vi "SetGas.vi"(7 "Timeout (ms)":u32=2000, 8 "Error In":errorcluster, 10 "Gas":T1, 11 "Sierra M100 In":refnum<visa-resource-name>) -> (0 "Error Out":errorcluster, 2 "Set?":bool, 3 "Sierra M100 Out":refnum<visa-resource-name>)   [LabVIEW 2012, in "Sierra-M100.lvlib"]
doc: "This VI sets the gas to be used with the mass flow controller."
uses:
  Sierra-M100.lvlib
  Controls/Gas.ctl
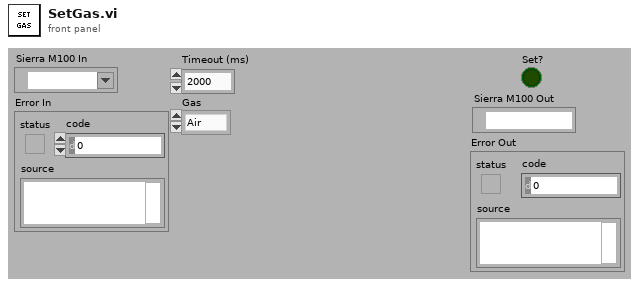
[diagram p1: front panel]
types:
  T1 = typedef "Sierra-M100.lvlib/Gas.ctl" = enum16{"Air", "Argon", "CO2", "CO", "Helium", "Hydrogen", "Methane", "Nitrogen", "Nitrous Oxide", "Oxygen"}
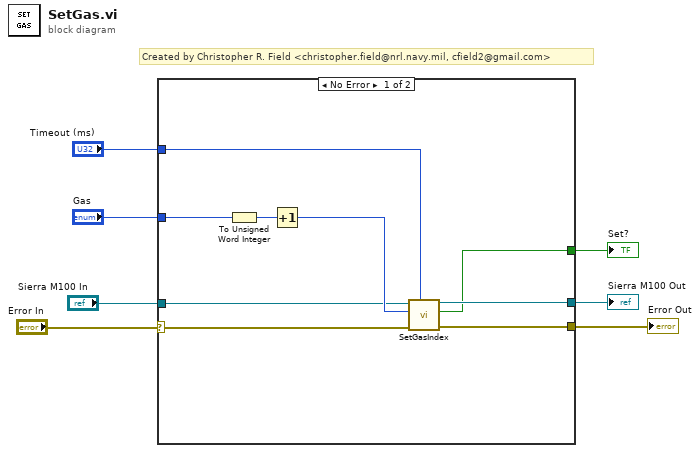
[diagram p0: block diagram]
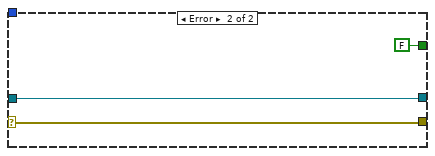
[diagram p2: hidden frame]
diagram:
  # "Created by Christopher R. Field <christopher.field@nrl.navy.mil, cfield2@gmail.com>"
  n1 = case shown="No Error" "Error In" {
    selector: "Error In" -> [w8 w18]
    tunnel: "Sierra M100 In" -> [w14 w19]
    tunnel: [w13 w19] -> w6
    tunnel: [w12 w18] -> w5
    tunnel: "Timeout (ms)" -> [w11 _]
    tunnel: [w10 FALSE ("Set?")] -> w3
    tunnel: "Gas" -> [w9 _]
    frame No Error {
      n2 = To Unsigned Word Integer(number=w9) -> (unsigned 16bit integer=w16:u16)
      n3 = Increment(x=w16) -> (x+1=w15:u16)
      n4 = call "SetGasIndex.vi"("Timeout (ms)"=w11, "Error In"=w8, "Gas Index"=w15, "Sierra M100 In"=w14) -> ("Error Out"=w12:errorcluster, "Set?"=w10:bool, "Sierra M100 Out"=w13:refnum<visa-resource-name>)  [unwired: 5 in]
    }
    frame Error {
    }
  }
  "Sierra M100 Out" <- w6
  "Error Out" <- w5
  "Set?" <- w3
